vi "Unpack For Grpc.vi"(8 "error in (no error)":errorcluster, 9 "Configuration / Resuls (Config)":enum16{"Configuration", "Results"}(ring), 10 "Any":T1, 11 "Measurement Customizations in":refnum<class "MeasurementPlugin.lvclass">) -> (0 "error out":errorcluster, 2 "Data Value":variant, 3 "Measurement Customizations out":refnum<class "MeasurementPlugin.lvclass">)   [LabVIEW 2021, in "adc_acMeasurement.lvlib" / "MeasurementPlugin.lvclass"]
uses:
  MeasurementPlugin.lvclass
  MeasurementPlugin.lvclass/MeasurementPlugin.ctl
  Measurement Configuration.ctl
  adc_acMeasurement.lvlib
  Measurement Results.ctl
  3ecd018e-d556-4cbc-bc60-c4ba57204520.vi
  a521b266-ce99-437c-923d-067dcf1e07fd.vi
  <vilib>/MeasurementLink/MeasurementLink Measurement Server/Measurement Plugin Service/Measurement Plugin Service.lvclass
  C:/Program Files/National Instruments/LabVIEW 2021/vi.lib/MeasurementLink/MeasurementLink Measurement Server/Measurement Plugin Service/Measurement Plugin Service.lvclass
  C:/Users/ksaravan/Documents/GitHub/data-converter-validation-module/source/measurements/ac/adc_acMeasurement/Advanced/MeasurementPlugin.lvclass
  <vilib>/gRPC/LabVIEW gRPC Library/Shared/Any.ctl
  <vilib>/gRPC/LabVIEW gRPC Library/grpc-lvsupport-release.lvlib
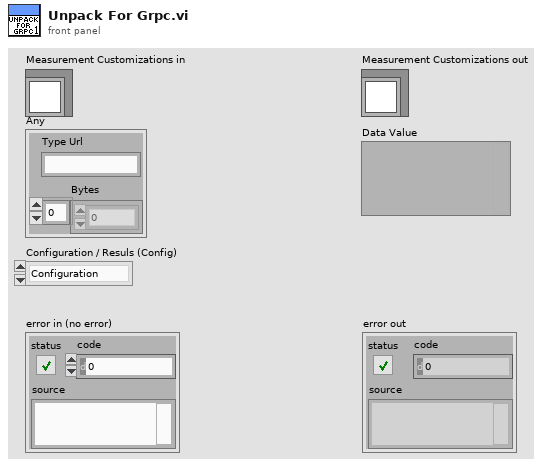
[diagram p1: front panel]
types:
  T1 = typedef "grpc-lvsupport-release.lvlib/Any.ctl" = cluster{"Type Url":string, "Bytes":u8[]}
  T2 = typedef "grpc-lvsupport-release.lvlib/grpcId.ctl" = u64
  T3 = typedef "adc_acMeasurement.lvlib/Measurement Configuration.ctl" = cluster{"Input channel":i32, "Full scale range":dbl, "Analog source resource name":string, "Frequency":dbl, "Amplitude":dbl, "Digital capture resource name":string, "Digital capture sample rate":dbl, "Digital capture samples":u32}
  T4 = typedef "adc_acMeasurement.lvlib/Measurement Results.ctl" = cluster{"Channel name":string, "Calculated frequency":dbl, "Calculated amplitude":dbl, "SNR":dbl, "THD":dbl, "SINAD":dbl, "SFDR":dbl, "ENOB":dbl, "f0":dbl, "df":dbl, "Spectrum":dbl[], "t0":dbl, "dt":dbl, "Time domain":dbl[]}
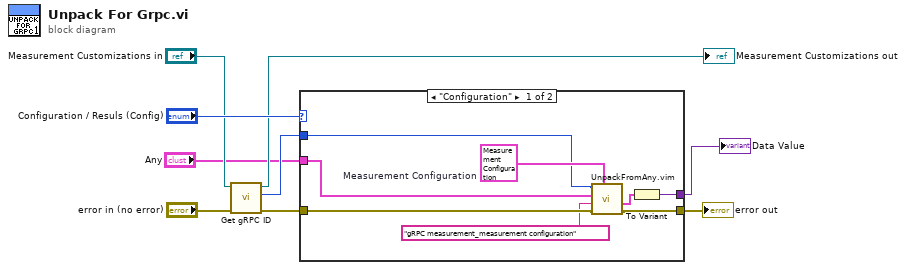
[diagram p0: block diagram]
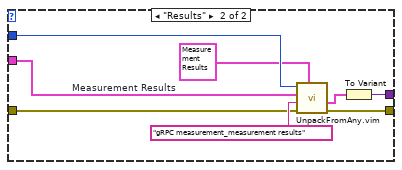
[diagram p2: hidden frame]
diagram:
  n1 = call <vilib>:"Get gRPC ID.vi"("error in"="error in (no error)", "measurement plugin service in"="Measurement Customizations in") -> ("error out"=w6:errorcluster, "gRPC ID"=w3:T2, "measurement plugin service out"=→"Measurement Customizations out":refnum<class "MeasurementPlugin.lvclass">)  [unwired: 7 in]
  n2 = case shown="\"Configuration\"" "Configuration / Resuls (Config)" {
    tunnel: w6 -> [w15 w19]
    tunnel: "Any" -> [w10 w18]
    tunnel: w3 -> [w12 w22]
    tunnel: [w16 w23] -> w9
    tunnel: [w17 w25] -> w1
    frame "Configuration" {
      w13 = T3 {"Input channel"=0, "Full scale range"=10.0, "Analog source resource name"="", "Frequency"=1000.0, "Amplitude"=-1.0, "Digital capture resource name"="", "Digital capture sample rate"=800000.0, "Digital capture samples"=800000}  # Measurement Configuration
      n3 = call "UnpackFromAny.vim"("Data Type"=w13, "error in"=w15, "Message Type"="gRPC measurement_measurement configuration", "Any"=w10, "gRPCid in"=w12) -> ("error out"=w16:errorcluster, "Unpacked Value"=w14:T3)  [unwired: 4 in, 1 out]
      n4 = To Variant(anything=w14) -> (Variant=w17:variant)
    }
    frame "Results" {
      w21 = T4 {"Channel name"="", "Calculated frequency"=0.0, "Calculated amplitude"=0.0, "SNR"=0.0, "THD"=0.0, "SINAD"=0.0, "SFDR"=0.0, "ENOB"=0.0, "f0"=0.0, "df"=0.0, "Spectrum"=[], "t0"=0.0, "dt"=0.0, "Time domain"=[]}  # Measurement Results
      n5 = call "UnpackFromAny.vim"("Data Type"=w21, "error in"=w19, "Message Type"="gRPC measurement_measurement results", "Any"=w18, "gRPCid in"=w22) -> ("error out"=w23:errorcluster, "Unpacked Value"=w24:T4)  [unwired: 4 in, 1 out]
      n6 = To Variant(anything=w24) -> (Variant=w25:variant)
    }
  }
  "error out" <- w9
  "Data Value" <- w1
